vi "Write position, mm.vi"(8 "error in (no error)":errorcluster, 9 "axis":i16, 10 "position, mm":dbl, 11 "DelayLineSimulation in":refnum<class "DLEmulate.lvclass">) -> (0 "error out":errorcluster, 3 "DelayLineSimulation out":refnum<class "DLEmulate.lvclass">)   [LabVIEW 2020, in "DLEmulate.lvclass"]
uses:
  DLEmulate.lvclass
  DLEmulate.lvclass/DLEmulate.ctl
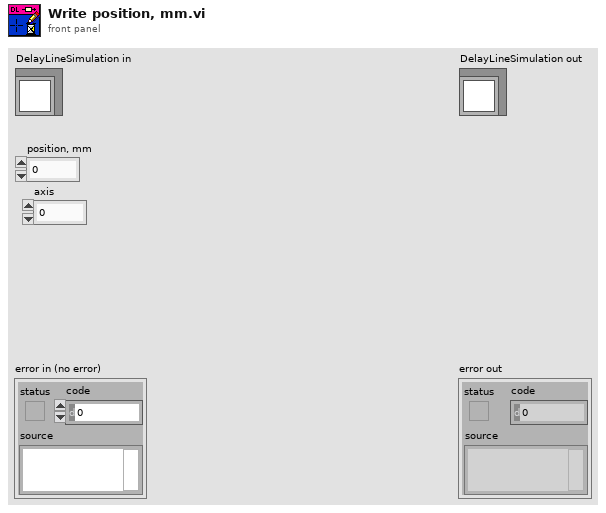
[diagram p1: front panel]
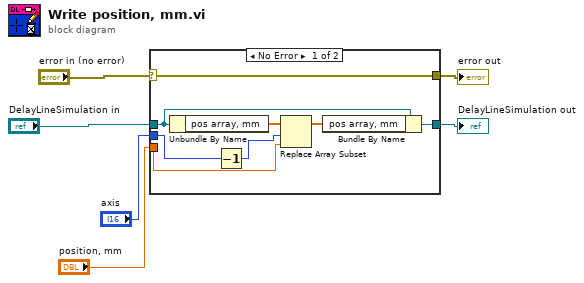
[diagram p0: block diagram]
diagram:
  n1 = case shown="No Error" "error in (no error)" {
    selector: "error in (no error)" -> [w14 w15]
    tunnel: [w14 w15] -> w5
    tunnel: [w13 w16] -> w3
    tunnel: "DelayLineSimulation in" -> [w12 w16]
    tunnel: "position, mm" -> [w8 _]
    tunnel: "axis" -> [w10 _]
    frame No Error {
      n2 = Unbundle By Name(w12) -> ("pos array, mm"=w11:dbl[])
      n3 = Decrement(x=w10) -> (x-1=w7:i16)
      n4 = Replace Array Subset(array=w11, new element=w8, index=w7) -> (w9:dbl[])
      n5 = Bundle By Name(cluster=w12, "pos array, mm"=w9) -> (w13:refnum<class "DLEmulate.lvclass">)
    }
    frame Error {
    }
  }
  "error out" <- w5
  "DelayLineSimulation out" <- w3
